vi "read_write_txt.vi"() -> ()   [LabVIEW 2010]
panel:
  in  "stop":bool
  in  "?":enum32{"Path", "Refnum"}(tab)
  in  "Write":string
  in  "Choose":string(combo)
  in  "Path":path
  out "Read Text":string
  in  "Path 2":path
  in  "Choose 2":string(combo)
  in  "Write":string
  out "Read":string
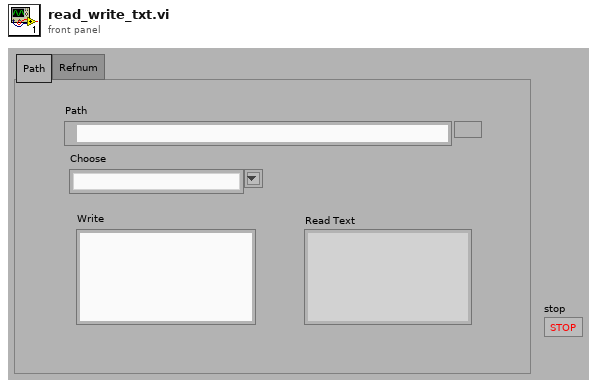
[diagram p1: front panel]
types:
  T1 = enum16{"open", "replace", "create", "open or create", "replace or create", "replace or create with confirmation"}
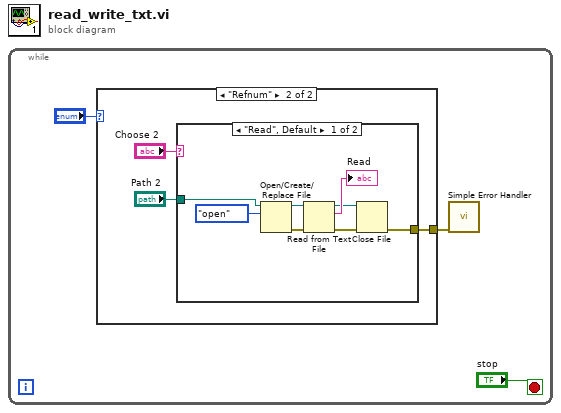
[diagram p0: block diagram]
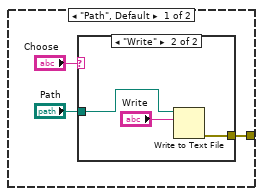
[diagram p2: hidden frame]
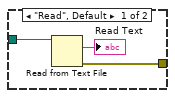
[diagram p3: hidden frame]
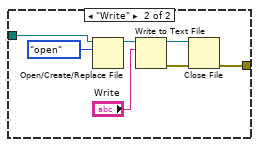
[diagram p4: hidden frame]
diagram:
  n1 = while {
    stop <- "stop" stop-if-true
    n2 = case shown="\"Refnum\"" "?" {
      tunnel: [w4 w13] -> w2
      frame "Path", Default {
        n3 = case shown="\"Write\"" "Choose" {
          tunnel: "Path" -> [w9 w12]
          tunnel: [w7 w10] -> w4
          frame "Read", Default {
            n4 = Read from Text File(file (use dialog)=w9) -> (text=→"Read Text":string, error out=w7:errorcluster)  [unwired: 3 in, 2 out]
          }
          frame "Write" {
            n5 = Write to Text File(file (use dialog)=w12, text="Write") -> (error out=w10:errorcluster)  [unwired: 2 in, 2 out]
          }
        }
      }
      frame "Refnum" {
        n6 = case shown="\"Read\", Default" "Choose 2" {
          tunnel: "Path 2" -> [w23 w30]
          tunnel: [w16 w24] -> w13
          frame "Read", Default {
            n7 = Open/Create/Replace File(file path (use dialog)=w23, operation (0:open)=T1."open") -> (refnum out=w21:refnum<file>, error out=w20:errorcluster)  [unwired: 4 in, 1 out]
            n8 = Read from Text File(file (use dialog)=w21, error in=w20) -> (refnum out=w17:refnum<file>, text=→"Read":string, error out=w18:errorcluster)  [unwired: 2 in, 1 out]
            n9 = Close File(refnum=w17, error in=w18) -> (error out=w16:errorcluster)  [unwired: 1 out]
          }
          frame "Write" {
            n10 = Open/Create/Replace File(file path (use dialog)=w30, operation (0:open)=T1."open") -> (refnum out=w28:refnum<file>)  [unwired: 4 in, 2 out]
            n11 = Write to Text File(file (use dialog)=w28, text="Write") -> (refnum out=w26:refnum<file>, error out=w25:errorcluster)  [unwired: 2 in, 1 out]
            n12 = Close File(refnum=w26, error in=w25) -> (error out=w24:errorcluster)  [unwired: 1 out]
          }
        }
      }
    }
    n13 = call <vilib>:"Simple Error Handler.vi"("error in (no error)"=w2) -> ()  [unwired: 4 in, 5 out]
  }
